vi "Test_ControlCaptionBinding_ValueOK.vi"(8 "error in (no error)":errorcluster, 11 "TestCase in":refnum<class "TestTransport.lvclass">) -> (0 "error out":errorcluster, 3 "TestCase out":refnum<class "TestTransport.lvclass">)   [LabVIEW 2017, in "TestTransport.lvclass"]
uses:
  TestTransport.lvclass
  Source/Framework/Transport/ControlCaptionBinding/ControlCaptionBinding.lvclass
panel:
  out "Button":bool caption="Caption!"
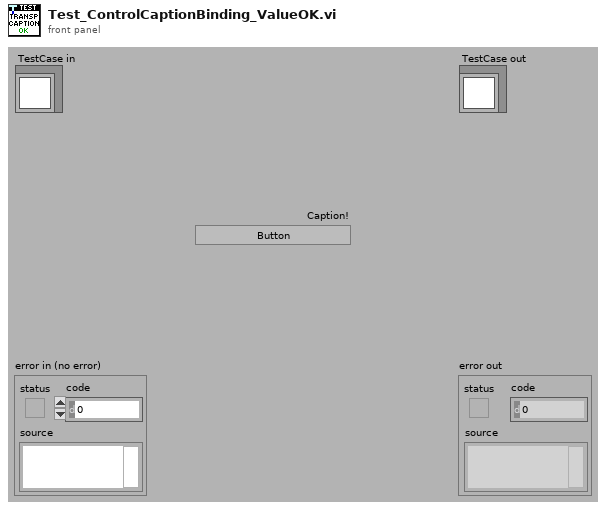
[diagram p1: front panel]
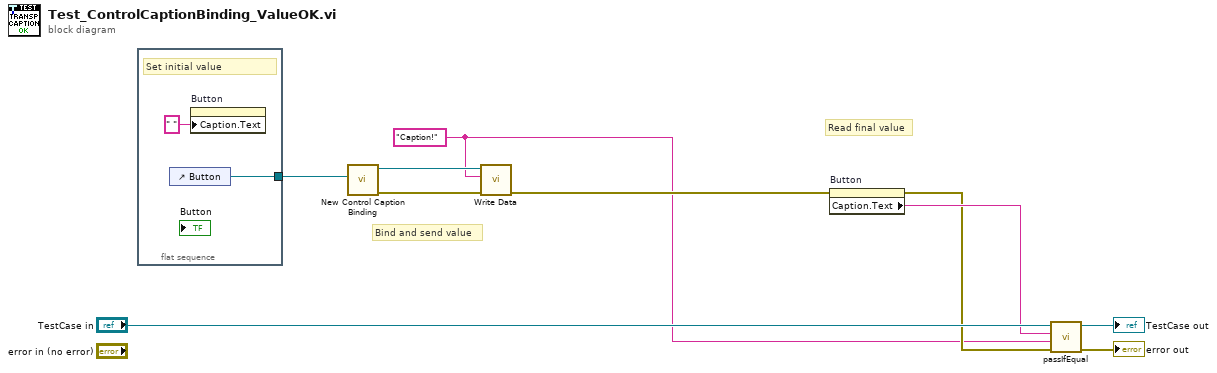
[diagram p0: block diagram]
diagram:
  w1 = "Caption!"
  # "Bind and send value"
  # "Read final value"
  n1 = flat-sequence {
    tunnel: [w12] -> w4
    frame #0 {
      # "Set initial value"
      n2 = control-ref of="Button"() -> (w12:refnum<vi>)
      n3 = property on="Button" class="Bool"("Caption.Text"=" " ("Boolean Text.Text")) -> ()  [unwired: 2 in, 2 out]
    }
  }
  n4 = call "New Control Caption Binding.vi"("Ctl Refnum"=w4) -> ("error out"=w3:errorcluster, "ControlCaptionBinding"=w6:refnum<class "ControlCaptionBinding.lvclass">)  [unwired: 9 in]
  n5 = call-dynamic "Write Data.vi"("error in (no error)"=w3, "Value"=w1, "ControlCaptionBinding in"=w6) -> ("error out"=w5:errorcluster)  [unwired: 7 in, 1 out]
  n6 = property on="Button" class="Bool"(error in=w5) -> (error out=w2:errorcluster, "Caption.Text"=w7:string)  [unwired: 1 in, 1 out]
  n7 = call-dynamic "passIfEqual.vi"("error in (no error)"=w2, "y"=w1, "x"=w7, "TestCase in"="TestCase in") -> ("error out"=→"error out":errorcluster, "TestCase out"=→"TestCase out":refnum<class "TestTransport.lvclass">)  [unwired: 6 in]
